vi "AnalogIn Read Value.vi"(7 "ADC #":T1=-1, 8 "error in (no error)":errorcluster, 11 "Session in":refnum<class "Session.lvclass">) -> (0 "error out":errorcluster, 2 "Value":T2, 3 "Session out":refnum<class "Session.lvclass">)   [LabVIEW 2020, in "CTI.lvlib" / "Session.lvclass"]
uses:
  Session.lvclass
  Session.lvclass/Session.ctl
  Raw ADC.ctl
  CTI.lvlib
  ADC Number.ctl
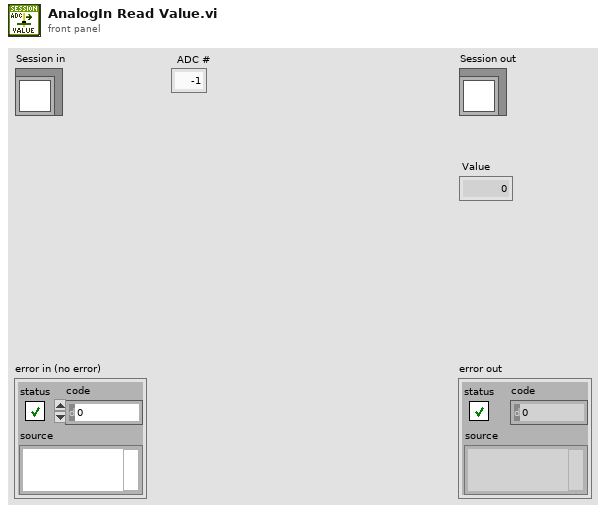
[diagram p1: front panel]
types:
  T1 = typedef "CTI.lvlib/ADC Number.ctl" = i8
  T2 = typedef "CTI.lvlib/Raw ADC.ctl" = u16
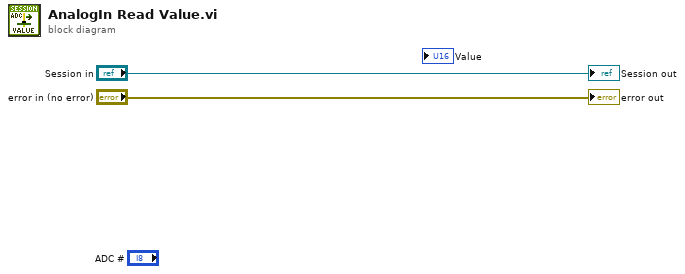
[diagram p0: block diagram]
diagram:
  "error out" <- "error in (no error)"
  "Session out" <- "Session in"
